vi "PRIVATE.ProcCases.vi"(0 "i ref in":refnum<vi>, 1 "selector":string, 2 "Data":T1, 3 "call cluster":T2={"Object"="", "Selector"="", "CallType"=enum."synchronous", "Async Object"="", "Async Selector"="", "Data Descriptor"="", "Data"=[], "Error #"=0, "Expire"=0}, 5 "error in (no error)":errorcluster) -> (14 "i ref out":refnum<vi>, 17 "answer cluster":T2={"Object"="", "Selector"="", "CallType"=enum."synchronous", "Async Object"="", "Async Selector"="", "Data Descriptor"="", "Data"=[], "Error #"=0, "Expire"=0}, 19 "error out":errorcluster)   [LabVIEW 2012]
doc: "This method is called by a process from within the default case in the event loop. The methods of a class that are linked to events will be called from THIS method. Add your code here."
uses:
  CSCore/CSSystem/CoreDefs/CoreDefs.call_type.ctl
  CSCore/BaseProcess/BaseProcess.descriptor string definition.ctl
  CSCore/CSSystem/CoreDefs/CoreDefs.rawDataType.ctl
  CSCore/CSSystem/CoreLib/CoreLib.byte array 2 double.vi
  CSCore/CSSystem/CoreLib/CoreLib.double 2 byte array.vi
  CSCore/CSSystem/CoreLib/CoreLib.string 2 byte array.vi
  CSCore/CSSystem/CoreLib/CoreLib.lvlib
  CSCore/BaseProcess/BaseProcess.lvlib
  CAEN_HVSystem.lvlib
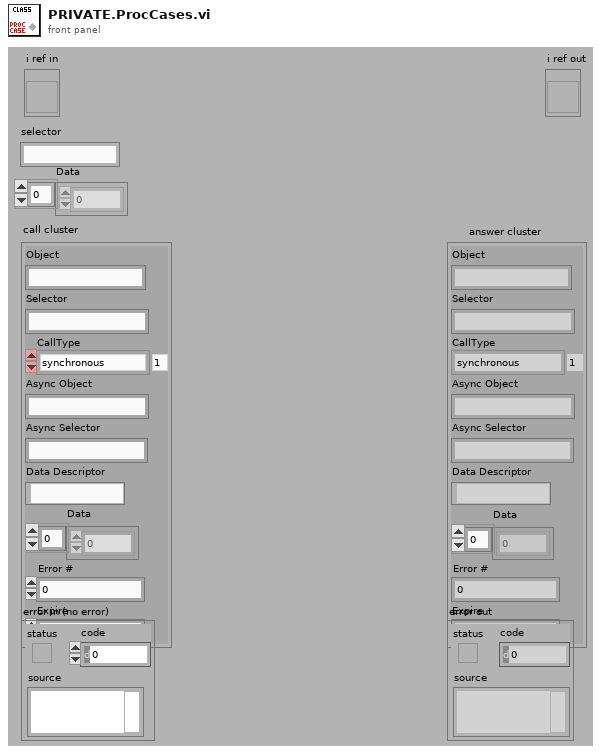
[diagram p1: front panel]
types:
  T1 = typedef "CoreDefs.rawDataType.ctl" = i8[]
  T2 = typedef "CoreDefs.call_type.ctl" = cluster{"Object":string, "Selector":string, "CallType":enum16{"simple", "synchronous", "asynchronous"}, "Async Object":string, "Async Selector":string, "Data Descriptor":T3, "Data":T1, "Error #":i32, "Expire":u32}
  T3 = typedef "BaseProcess.lvlib/BaseProcess.descriptor string definition.ctl" = string
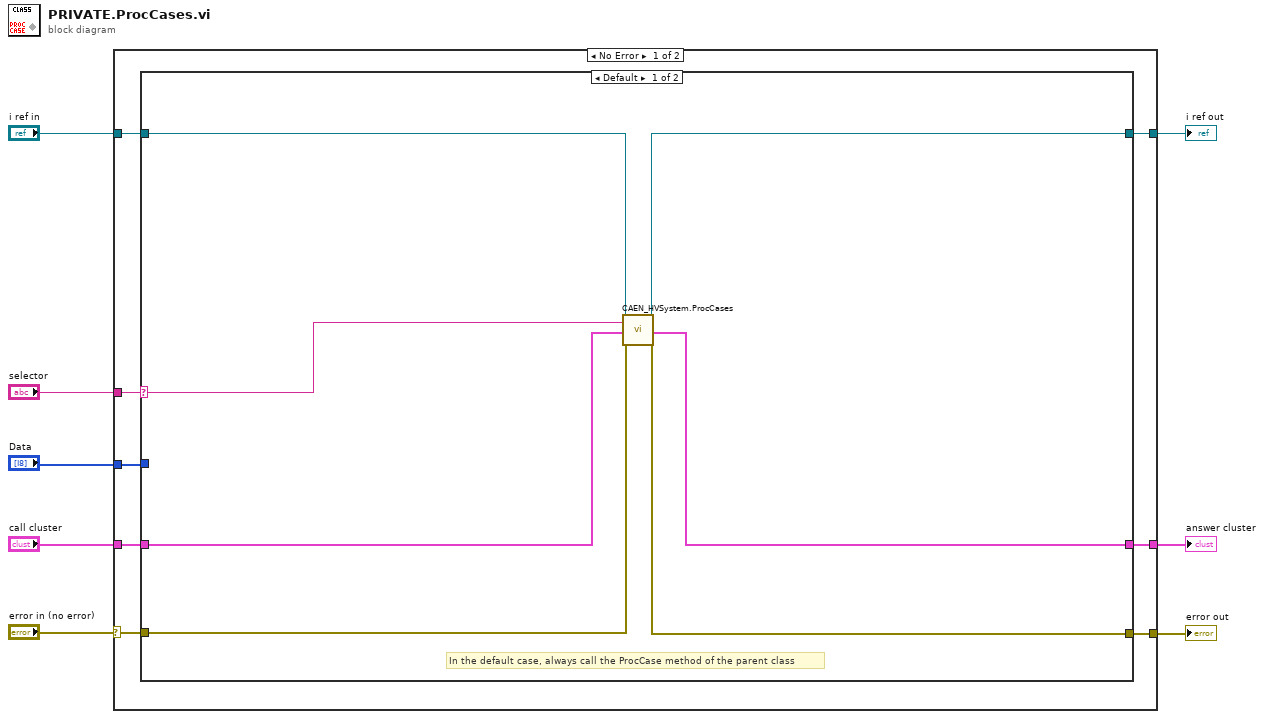
[diagram p0: block diagram]
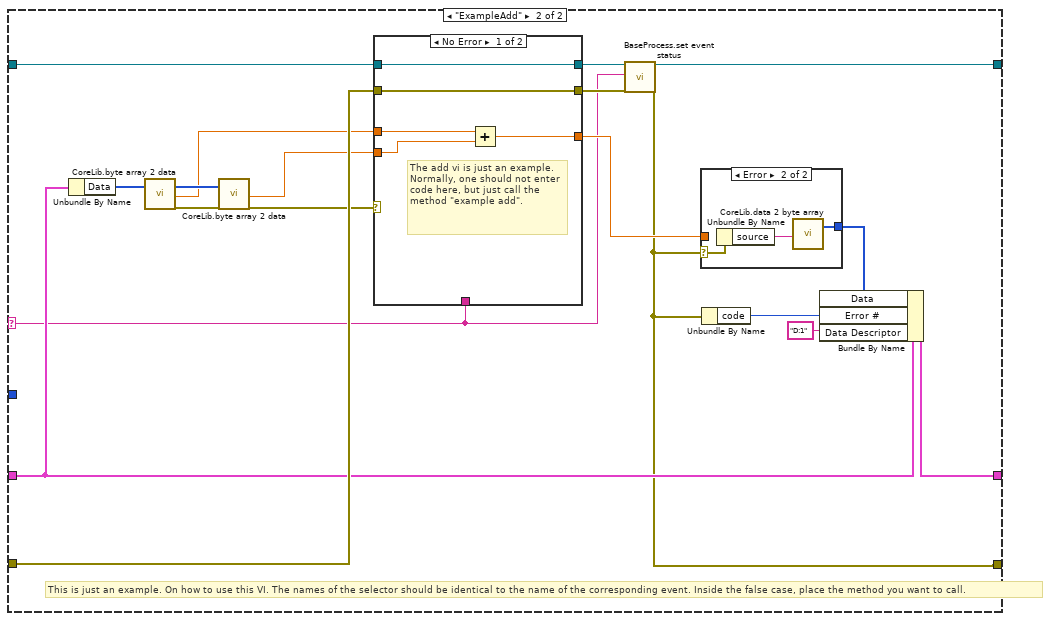
[diagram p2: hidden frame]
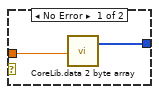
[diagram p3: hidden frame]
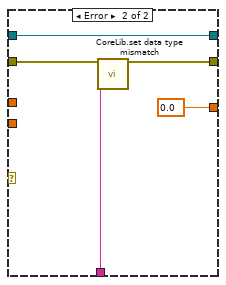
[diagram p4: hidden frame]
diagram:
  n1 = case shown="No Error" "error in (no error)" {
    selector: "error in (no error)" -> [w9 w58]
    tunnel: "selector" -> [w16 _]
    tunnel: [w15 w59] -> w7
    tunnel: "Data" -> [w14 _]
    tunnel: "call cluster" -> [w13 w59]
    tunnel: "i ref in" -> [w12 w60]
    tunnel: [w11 w60] -> w3
    tunnel: [w10 w58] -> w2
    frame No Error {
      n2 = case shown="Default" w16 {
        selector: w16 -> [w18 w32]
        tunnel: w14 -> [_ _]
        tunnel: w12 -> [w17 w42]
        tunnel: [w23 w31] -> w11
        tunnel: w13 -> [w19 w38]
        tunnel: [w20 w37] -> w15
        tunnel: w9 -> [w22 w41]
        tunnel: [w21 w33] -> w10
        frame Default {
          # "In the default case, always call the ProcCase method of the parent class"
          n3 = call "CAEN_HVSystem.ProcCases.vi"("i ref in"=w17, "selector"=w18, "call cluster"=w19, "error in (no error)"=w22) -> ("i ref out"=w23:refnum<vi>, "answer cluster"=w20:T2, "error out"=w21:errorcluster)  [unwired: 13 in]
        }
        frame "ExampleAdd" {
          # "This is just an example. On how to use this VI. The names of the selector should be identical to the name of the corresponding event. Inside the false case, place the method you want to call."
          n4 = Unbundle By Name(w38) -> ("Data"=w29:T1)
          n5 = call-poly "CoreLib.byte array 2 data.vi"("byteArray"=w29) -> ("byteArray out"=w27:T1, "d64"=w25:dbl, "error out"=w28:errorcluster)  [unwired: 16 in]
          n6 = call-poly "CoreLib.byte array 2 data.vi"("byteArray"=w27, "error in (no error)"=w28) -> ("d64"=w24:dbl, "error out"=w26:errorcluster)  [unwired: 15 in, 1 out]
          n7 = case shown="No Error" w26 {
            tunnel: [w49 w57] -> w35
            tunnel: w42 -> [w49 w57]
            tunnel: w41 -> [w50 w56]
            tunnel: [w50 w55] -> w34
            tunnel: w24 -> [w52 _]
            tunnel: [w51 0.0] -> w40
            tunnel: w32 -> [_ w53]
            tunnel: w25 -> [w48 _]
            frame No Error {
              # "The add vi is just an example. Normally, one should not enter code here, but just call the method \"example add\"."
              n8 = Add(x=w48, y=w52) -> (x+y=w51:dbl)
            }
            frame Error {
              n9 = call "CoreLib.set data type mismatch.vi"("error in (no error)"=w56, "error source"=w53) -> ("error out"=w55:errorcluster)  [unwired: 17 in]
            }
          }
          n10 = call "BaseProcess.set event status.vi"("i ref in"=w35, "EventStatus"=w32, "error in (no error)"=w34) -> ("i ref out"=w31:refnum<vi>, "error out"=w33:errorcluster)  [unwired: 14 in, 1 out]
          n11 = case shown="Error" w33 {
            selector: w33 -> [_ w47]
            tunnel: [w43 w46] -> w36
            tunnel: w40 -> [w44 _]
            frame No Error {
              n12 = call-poly "CoreLib.data 2 byte array.vi"("f64"=w44) -> ("byteArray out"=w43:T1)  [unwired: 18 in]
            }
            frame Error {
              n13 = Unbundle By Name(w47) -> ("source"=w45:string)
              n14 = call-poly "CoreLib.data 2 byte array.vi"("string"=w45) -> ("byteArray out"=w46:T1)  [unwired: 18 in]
            }
          }
          n15 = Unbundle By Name(w33) -> ("code"=w39:i32)
          n16 = Bundle By Name(cluster=w38, "Data"=w36, "Error #"=w39, "Data Descriptor"="D:1") -> (w37:T2)
        }
      }
    }
    frame Error {
    }
  }
  "answer cluster" <- w7
  "i ref out" <- w3
  "error out" <- w2
